vi "Setup.vi"(8 "error in":errorcluster, 11 "Fault_Engine in":refnum<class "Engine.lvclass">) -> (0 "error out":errorcluster, 3 "Fault_Engine out":refnum<class "Engine.lvclass">)   [LabVIEW 2019, in "Engine.lvlib" / "Engine.lvclass"]
doc: "Part of the instantiation process for every ancestor class. This routine interrogates the IsRoot Flag.\n\nIf this is the root actor, it reads its self enqueuer to memoury\n\nIf this is a nested actor, it reads its self enqueuer and the caller enqueuer to memory"
uses:
  Project/Engine.lvclass
  C:/Users/Public/Documents/Development/builds/Engine/Actor Framework.lvlibp/1abvi3w/vi.lib/ActorFramework/Actor/Actor.lvclass
  Project/Engine.lvclass/Engine.ctl
  builds/Engine/Actor Framework.lvlibp/1abvi3w/vi.lib/ActorFramework/Actor/Actor.lvclass
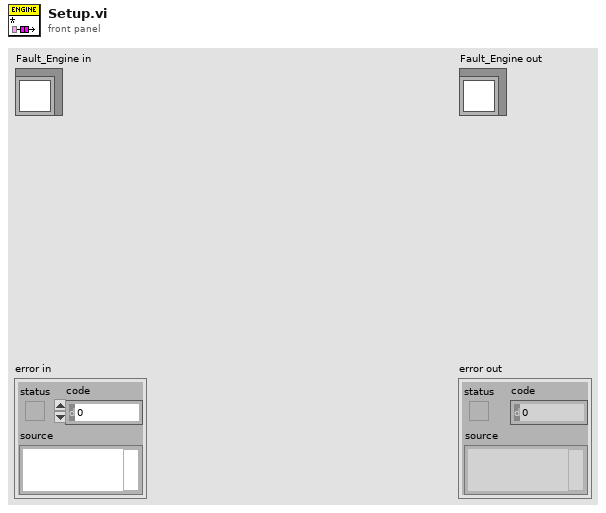
[diagram p1: front panel]
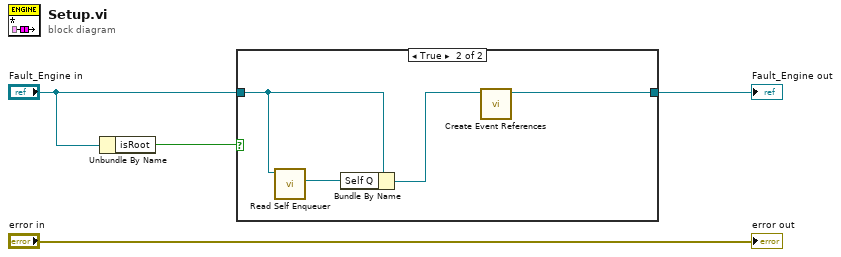
[diagram p0: block diagram]
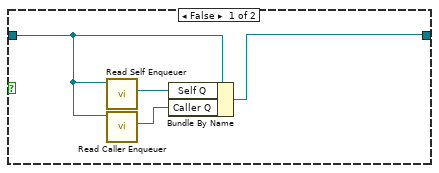
[diagram p2: hidden frame]
diagram:
  n1 = Unbundle By Name("Fault_Engine in") -> ("isRoot"=w4:bool)
  n2 = case shown="True" w4 {
    tunnel: "Fault_Engine in" -> [w8 w12]
    tunnel: [w7 w9] -> w2
    frame False {
      n3 = call "Read Self Enqueuer.vi"("Actor"=w8) -> ("Self Enqueuer"=w6:refnum<class "Message Enqueuer.lvclass">)  [unwired: 10 in]
      n4 = call "Read Caller Enqueuer.vi"("Actor"=w8) -> ("Caller Enqueuer"=w5:refnum<class "Message Enqueuer.lvclass">)  [unwired: 10 in]
      n5 = Bundle By Name(cluster=w8, "Self Q"=w6, "Caller Q"=w5) -> (w7:refnum<class "Engine.lvclass">)
    }
    frame True {
      n6 = call "Read Self Enqueuer.vi"("Actor"=w12) -> ("Self Enqueuer"=w11:refnum<class "Message Enqueuer.lvclass">)  [unwired: 10 in]
      n7 = Bundle By Name(cluster=w12, "Self Q"=w11) -> (w10:refnum<class "Engine.lvclass">)
      n8 = call "Create Event References.vi"("Engine in"=w10) -> ("Engine out"=w9:refnum<class "Engine.lvclass">)  [unwired: 9 in, 1 out]
    }
  }
  "Fault_Engine out" <- w2
  "error out" <- "error in"
